vi "hWrite2014.vi"(4 "error in":errorcluster, 5 "nbit":u8, 6 "Data":bool[](array[boolean])=[FALSE, FALSE, FALSE, FALSE, FALSE, FALSE, FALSE, FALSE, FALSE, FALSE, FALSE, FALSE, FALSE, FALSE, FALSE, FALSE, FALSE, FALSE, FALSE, FALSE, FALSE, FALSE, FALSE, FALSE, FALSE, FALSE, FALSE, FALSE, FALSE, FALSE, FALSE, FALSE], 7 "FPGA VI Reference In":refnum<k20>) -> (0 "error out":errorcluster, 2 "Timed Out":bool, 3 "FPGA VI Reference Out":refnum<k20>)   [LabVIEW 2014]
doc: "Übergibt an FPGA ein 32bit Array, wobei nbit ausgegeben werden.\nNach dem Schreiben wird auf IRQ3 gewartet(mit 2 ms Timeout).\nAdressierung muss vorher angelegt werden!"
uses:
  <vilib>/Utility/error.llb/Error Cluster From Error Code.vi
  <vilib>/rvi/errors/niLvFpgaAdjustHostInterfaceError.vi
  <vilib>/RVI Host/nirviSupport.llb/nirviErrorClusterFromErrorCode.vi
  <vilib>/rvi/interface/nirviReadWriteControl/nirviReadWriteControl.xnode
  FPGA Bitfiles/W7XBolo2017_FPGATarget_FlorianDefault.lvbitx
  f_main_2014.vi
  <vilib>/rvi/interface/nirviMethod/nirviMethod.xnode
  NiFpgaLv.dll
  <vilib>/rvi/interface/nirviMethod/StockFPGA_InlinedMethodWaitForSingleIRQ.vi
  <vilib>/FPGAPlugInAG/PCI-7813R/niLvFpga_WaitOnIrq_PCI-7813R.vi
  <vilib>/FPGAPlugInAG/PCI-7813R/niLvFpga_AcknowledgeIrq_PCI-7813R.vi
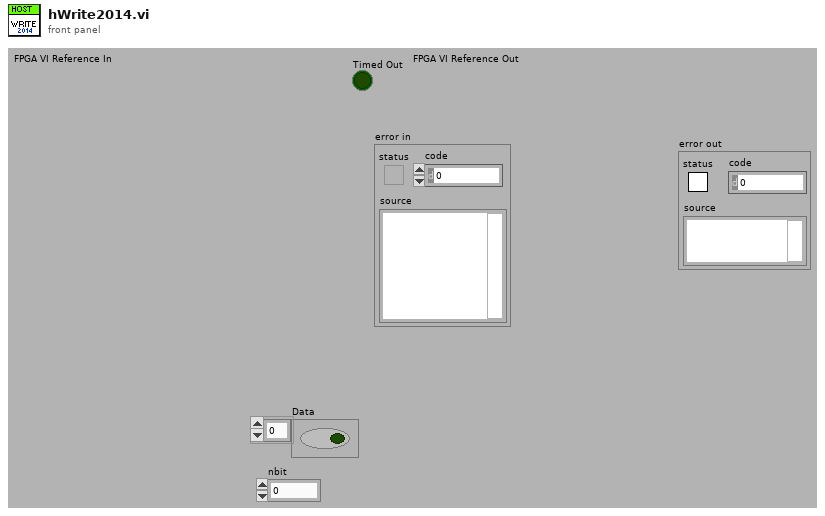
[diagram p1: front panel]
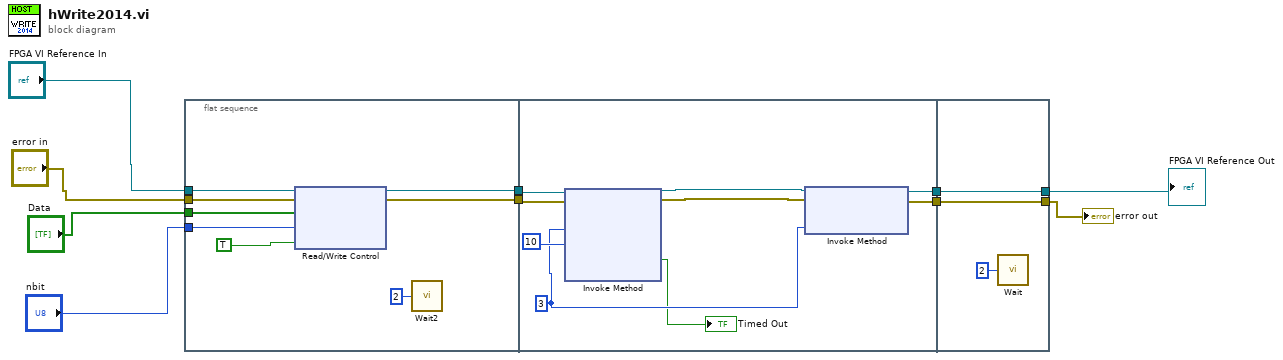
[diagram p0: block diagram]
diagram:
  n1 = flat-sequence {
    tunnel: "nbit" -> [w18]
    tunnel: "error in" -> [w17]
    tunnel: "FPGA VI Reference In" -> [w16]
    tunnel: "Data" -> [w13]
    tunnel: [w15] -> w10
    tunnel: [w14] -> w9
    tunnel: w10 -> [w24]
    tunnel: w9 -> [w25]
    tunnel: [w27] -> w5
    tunnel: [w26] -> w4
    tunnel: [w29] -> w3
    tunnel: [w30] -> w2
    tunnel: w5 -> [w30]
    tunnel: w4 -> [w29]
    frame #0 {
      n2 = xnode "Read/Write Control"("FPGA VI Reference In"=w16, "error in"=w17, "Serial Data Out"=w13, "nbit"=w18, "SPIWrite"=TRUE) -> ("FPGA VI Reference Out"=w14:refnum<k20>, "error out"=w15:errorcluster)
      n3 = call "Wait2"("Count(mSec)"=u32 2) -> ()  [unwired: 1 out]
    }
    frame #1 {
      w22 = 3 ("IRQ Number(s)")
      n4 = xnode "Invoke Method"("FPGA VI Reference In"=w25, "error in"=w24, "IRQ Number(s)"=w22, "Timeout (ms)"=10 ("timeout (ms)(-1 for no timeout)")) -> ("FPGA VI Reference Out"=w19:refnum<k20>, "error out"=w20:errorcluster, "Timed Out"=→"Timed Out":bool)  [unwired: 1 out]
      n5 = xnode "Invoke Method"("FPGA VI Reference In"=w19, "error in"=w20, "IRQ Number(s)"=w22) -> ("FPGA VI Reference Out"=w27:refnum<k20>, "error out"=w26:errorcluster)
    }
    frame #2 {
      n6 = call "Wait"("Count(mSec)"=u32 2 ("milliseconds to wait")) -> ()  [unwired: 1 out]
    }
  }
  "error out" <- w3
  "FPGA VI Reference Out" <- w2
